vi "Reset Label Strings.vi"(4 "Tick Array":T2, 5 "Right justified":bool, 6 "Range":cluster{"Max X":sgl, "Min X":sgl}, 7 "Which Axis?":T1(ring)=enum."Z Opposite", 8 "error in (no error)":errorcluster, 9 "Inverted?":bool, 10 "Size":u16, 11 "Axis Scene Object in":refnum<vi>) -> (0 "error out":errorcluster, 3 "Axis Scene Object out":refnum<vi>)   [LabVIEW 2017, in "3D Plot.lvclass"]
uses:
  <vilib>/Math Plots/3D Math Plots/3D Plot/3D Plot/3D Plot.lvclass
  <vilib>/Math Plots/3D Math Plots/3D Plot/3D Plot/Typedef/Tick Array.ctl
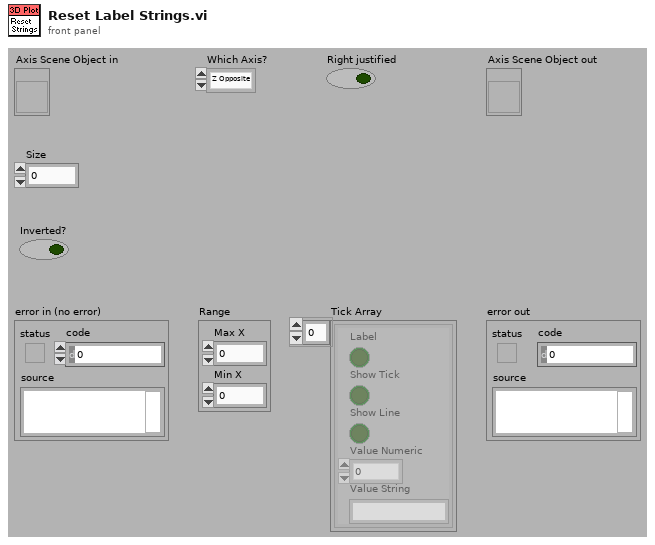
[diagram p1: front panel]
types:
  T1 = enum16{"X", "Y", "Z", "X Opposite", "Y Opposite", "Z Opposite"}
  T2 = typedef "3D Plot.lvclass/Tick Array.ctl" = cluster{"Label":bool, "Show Tick":bool, "Show Line":bool, "Value Numeric":sgl, "Value String":string}[]
  T3 = typedef "LVRGBAColorTypeDef.ctl" = cluster{"Red":sgl, "Green":sgl, "Blue":sgl, "Alpha":sgl}
  T4 = typedef "LV3DPointTypeDef.ctl" = cluster{"X":sgl, "Y":sgl, "Z":sgl}
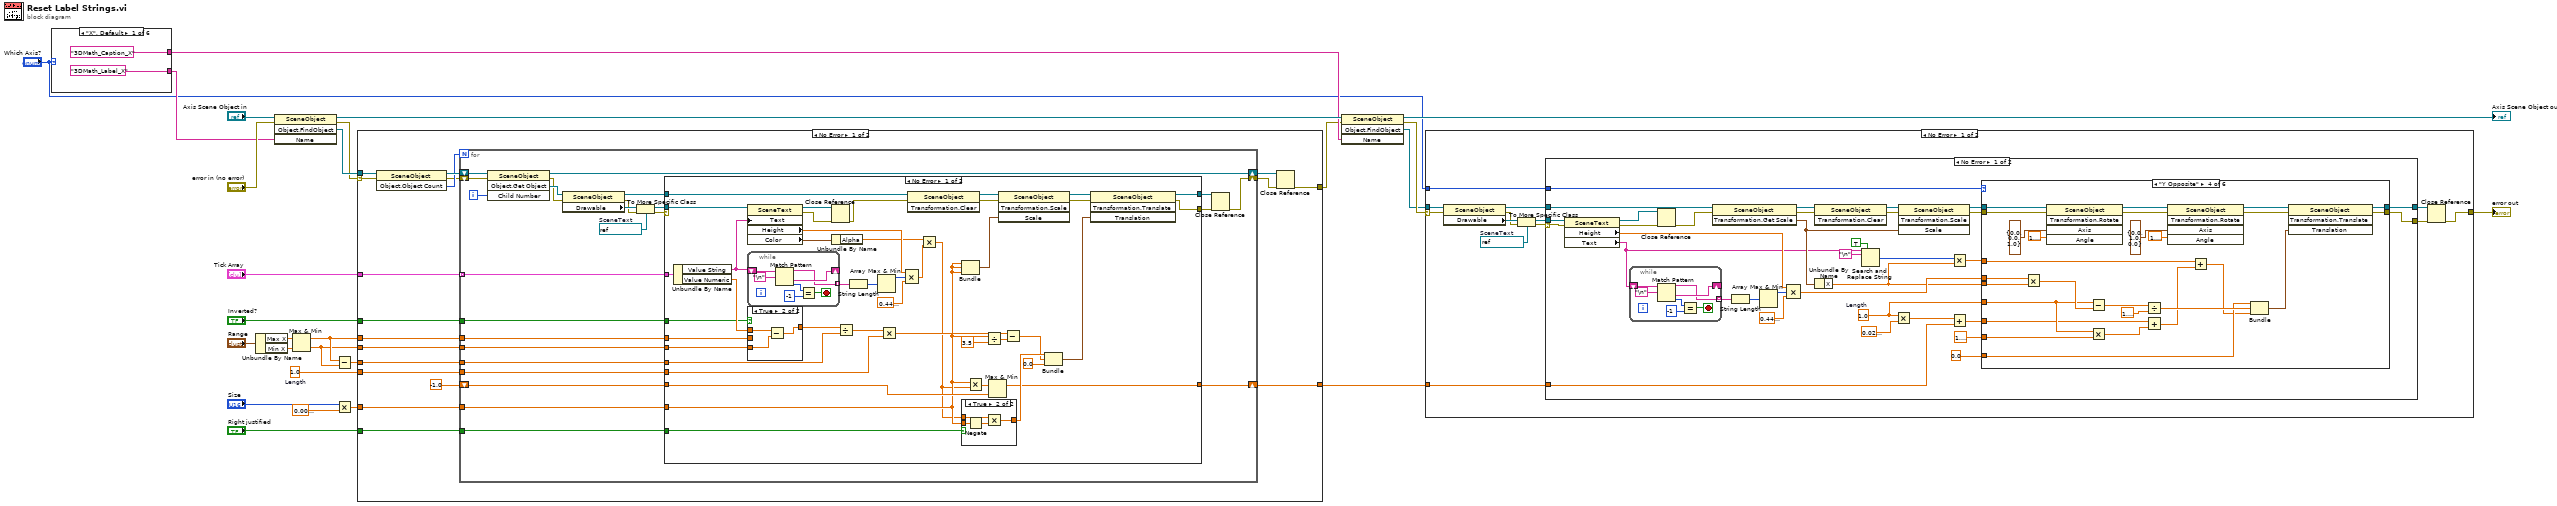
[diagram p0: block diagram]
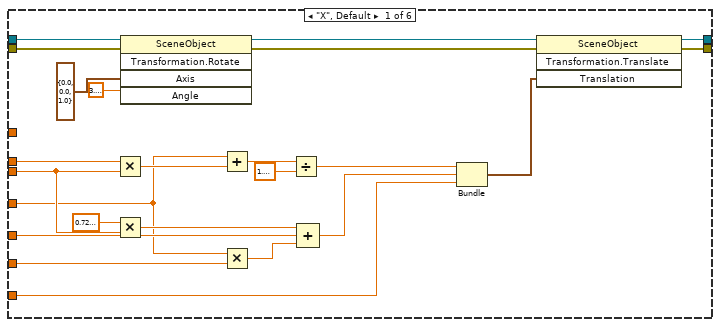
[diagram p2: hidden frame]
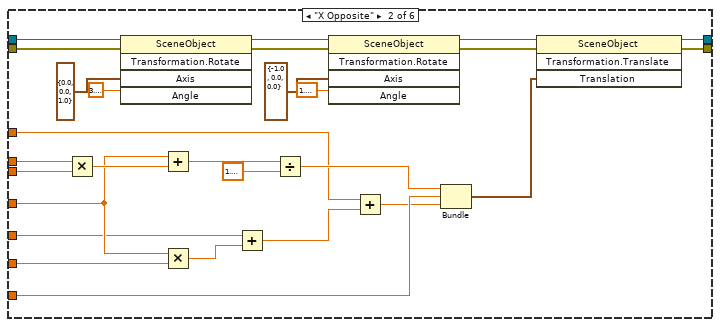
[diagram p3: hidden frame]
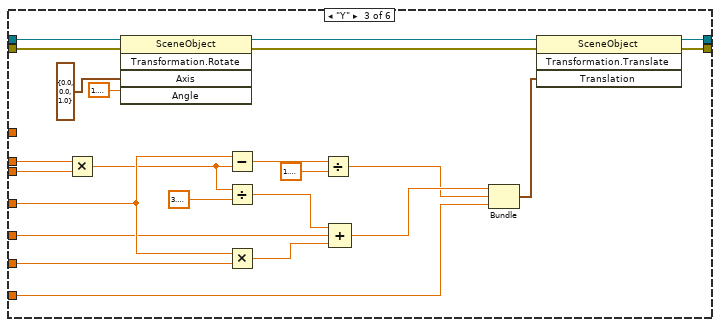
[diagram p4: hidden frame]
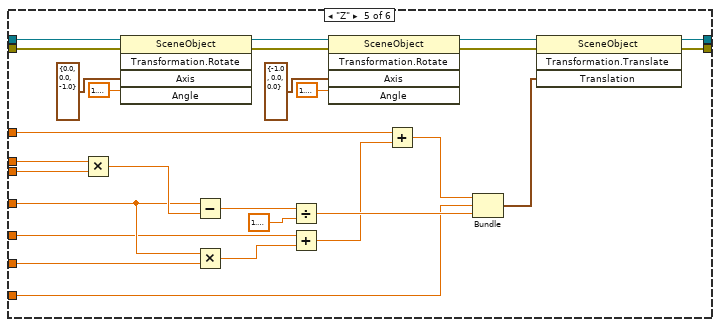
[diagram p5: hidden frame]
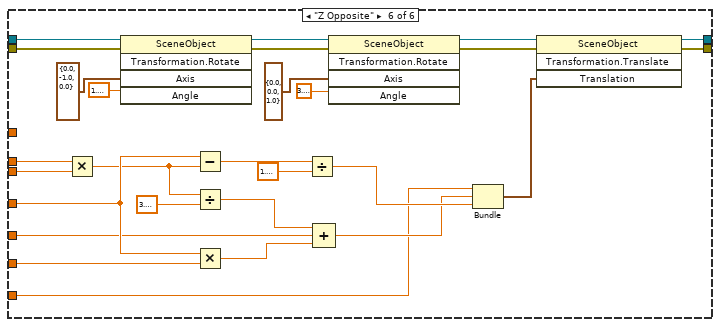
[diagram p6: hidden frame]
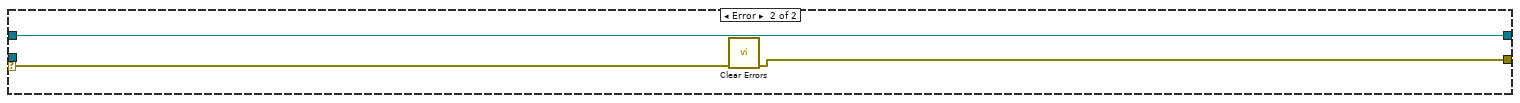
[diagram p7: hidden frame]
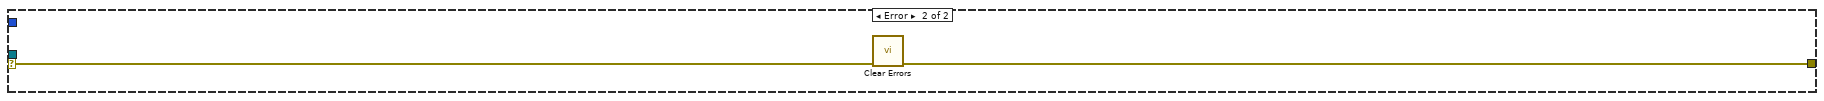
[diagram p8: hidden frame]
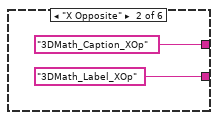
[diagram p9: hidden frame]
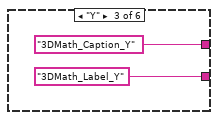
[diagram p10: hidden frame]
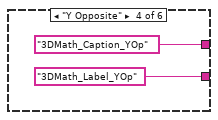
[diagram p11: hidden frame]
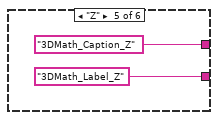
[diagram p12: hidden frame]
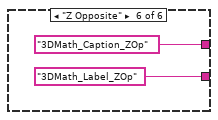
[diagram p13: hidden frame]
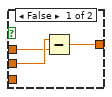
[diagram p14: hidden frame]
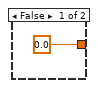
[diagram p15: hidden frame]
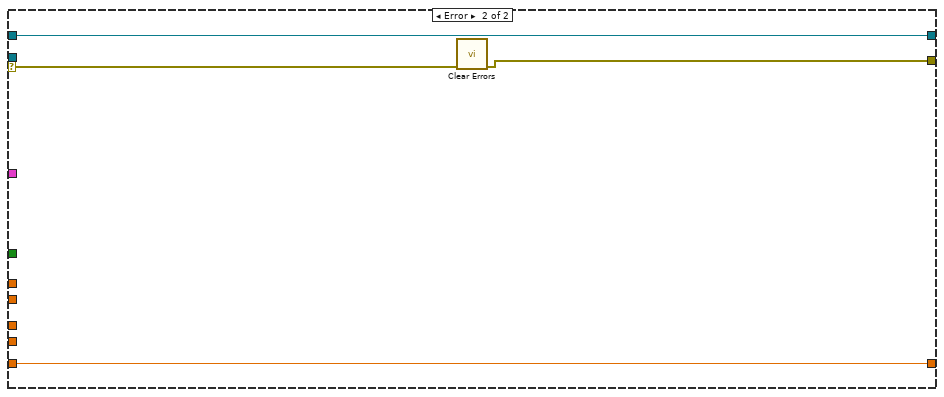
[diagram p16: hidden frame]
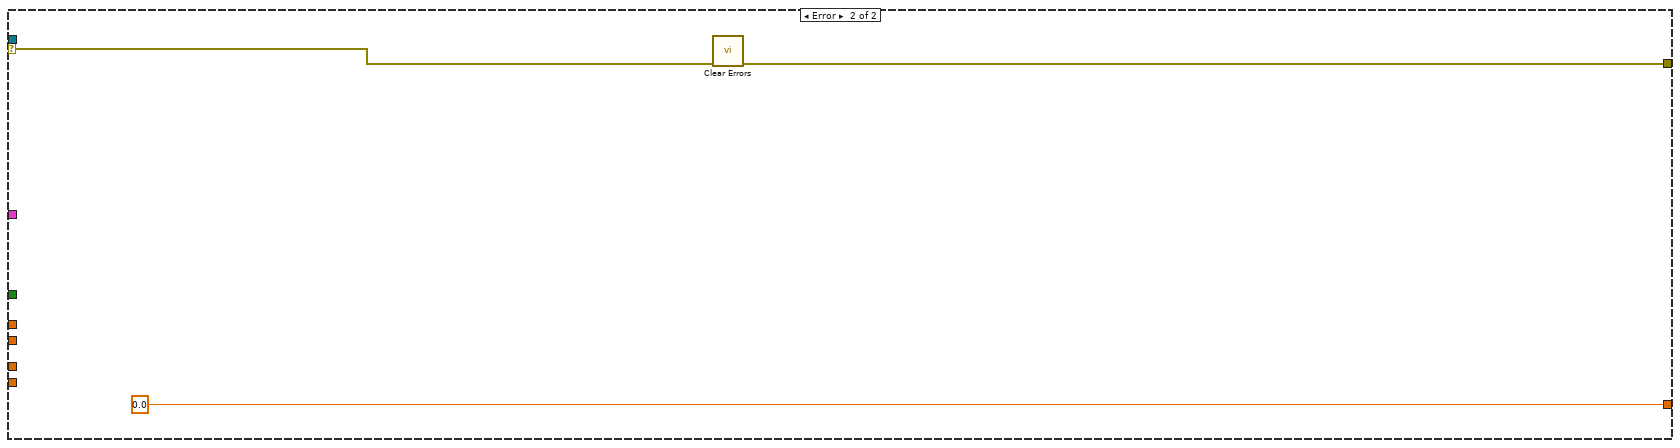
[diagram p17: hidden frame]
diagram:
  w11 = sgl 1.0  # Length
  n1 = case shown="\"X\", Default" "Which Axis?" {
    tunnel: ["3DMath_Label_X" ("Label Object Name") "3DMath_Label_XOp" ("Label Object Name") "3DMath_Label_Y" ("Label Object Name") "3DMath_Label_YOp" ("Label Object Name") "3DMath_Label_Z" ("Label Object Name") "3DMath_Label_ZOp" ("Label Object Name")] -> w9
    tunnel: ["3DMath_Caption_X" "3DMath_Caption_XOp" "3DMath_Caption_Y" "3DMath_Caption_YOp" "3DMath_Caption_Z" "3DMath_Caption_ZOp"] -> w7
    frame "X", Default {
    }
    frame "X Opposite" {
    }
    frame "Y" {
    }
    frame "Y Opposite" {
    }
    frame "Z" {
    }
    frame "Z Opposite" {
    }
  }
  n2 = Unbundle By Name("Range") -> ("Max X"=w18:sgl, "Min X"=w19:sgl)
  n3 = invoke class="SceneObject" method="Object.FindObject"(reference="Axis Scene Object in", error in="error in (no error)", "Name"=w9) -> (reference out=w24:refnum<vi>, error out=w22:errorcluster, "FindObject"=w23:refnum<vi>)  [unwired: 1 in, 1 out]
  n4 = Max & Min(x=w18, y=w19) -> (max(x,y)=w13:sgl, min(x,y)=w12:sgl)
  n5 = Subtract(x=w13, y=w12) -> (x-y=w15:sgl)
  n6 = Multiply(x="Size", y=sgl 0.01) -> (x*y=w10:sgl)
  n7 = case shown="No Error" w22 {
    selector: w22 -> [w57 w150]
    tunnel: w23 -> [w56 _]
    tunnel: [w49 w149] -> w4
    tunnel: "Tick Array" -> [w52 _]
    tunnel: w10 -> [w48 _]
    tunnel: "Right justified" -> [w47 _]
    tunnel: w11 -> [w46 _]
    tunnel: w15 -> [w45 _]
    tunnel: "Inverted?" -> [w44 _]
    tunnel: w13 -> [w43 _]
    tunnel: w12 -> [w42 _]
    tunnel: [w41 sgl 0.0] -> w1
    frame No Error {
      n8 = invoke class="SceneObject" method="Object.Object Count"(reference=w56, error in=w57) -> (reference out=w55:refnum<vi>, error out=w53:errorcluster, "Child Count"=w54:i32)  [unwired: 1 in]
      n9 = for {
        N: w54 -> [_]
        shift-right: [w73] -> w51
        shift-left: w53 -> [w80]
        tunnel: w52 -> [w61] mode=indexing
        shift-right: [w72] -> w50
        shift-left: w55 -> [w82]
        shift-right: [w67] -> w41
        shift-left: sgl -1.0 -> [w66]
        tunnel: w48 -> [w65]
        tunnel: w47 -> [w64]
        tunnel: w46 -> [w63]
        tunnel: w45 -> [w62]
        tunnel: w44 -> [w60]
        tunnel: w43 -> [w59]
        tunnel: w42 -> [w58]
        i -> [w81]
        w78 = refnum<vi> refnum  # SceneText
        n10 = invoke class="SceneObject" method="Object.Get Object"(reference=w82, error in=w80, "Child Number"=w81) -> (reference out=w72:refnum<vi>, error out=w70:errorcluster, "Get Child"=w71:refnum<vi>)  [unwired: 1 in, 1 out]
        n11 = property class="SceneObject"(reference=w71, error in=w70) -> (reference out=w69:refnum<vi>, error out=w76:errorcluster, "Drawable"=w79:refnum<vi>)
        n12 = To More Specific Class(target class=w78, reference=w79, error in=w76) -> (specific class reference=w77:refnum<vi>, error out=w75:errorcluster)
        n13 = case shown="No Error" w75 {
          selector: w75 -> [_ w147]
          tunnel: w77 -> [w123 _]
          tunnel: [w87 w146] -> w74
          tunnel: w69 -> [w94 w145]
          tunnel: [w116 w145] -> w68
          tunnel: [w105 w144] -> w67
          tunnel: w66 -> [w104 w144]
          tunnel: w65 -> [w92 _]
          tunnel: w64 -> [w103 _]
          tunnel: w63 -> [w102 _]
          tunnel: w62 -> [w101 _]
          tunnel: w61 -> [w99 _]
          tunnel: w60 -> [w97 _]
          tunnel: w59 -> [w96 _]
          tunnel: w58 -> [w95 _]
          frame No Error {
            n14 = Unbundle By Name(w99) -> ("Value String"=w100:string, "Value Numeric"=w98:sgl)
            n15 = property class="SceneText"(reference=w123, "Text"=w100) -> (reference out=w125:refnum<vi>, error out=w124:errorcluster, "Height"=w119:sgl, "Color"=w86:T3)  [unwired: 1 in]
            n16 = while {
              shift-right: [w142] -> _
              shift-left: w100 -> [w143]
              tunnel: [w141] -> w120 mode=indexing
              stop <- w139 stop-if-true
              n17 = Match Pattern(string=w143, regular expression="\n") -> (before substring=w141:string, after substring=w142:string, offset past match=w138:i32)  [unwired: 2 out]
              n18 = Equal?(x=w138, y=-1) -> (x = y?=w139:bool)
            }
            n19 = case shown="True" w97 {
              tunnel: [w128 w129] -> w109
              tunnel: w96 -> [w127 _]
              tunnel: w98 -> [w126 w131]
              tunnel: w95 -> [_ w130]
              frame False {
                n20 = Subtract(x=w127, y=w126) -> (x-y=w128:sgl)
              }
              frame True {
                n21 = Subtract(x=w131, y=w130) -> (x-y=w129:sgl)
              }
            }
            n22 = Close Reference(reference=w125, error in (no error)=w124) -> (error out=w90:errorcluster)
            n23 = Unbundle By Name(w86) -> ("Alpha"=w85:sgl)
            n24 = Divide(x=w109, y=w101) -> (x/y=w108:sgl)
            n25 = String Length(string=w120) -> (length=w121:i32[])
            n26 = Array Max & Min(array=w121) -> (max value=w91:i32)  [unwired: 3 out]
            n27 = Multiply(x=w108, y=w102) -> (x*y=w110:sgl)
            n28 = Compound Arithmetic op=MULTIPLY(w119, w91, sgl 0.45 ("y")) -> (w84:sgl)
            n29 = invoke class="SceneObject" method="Transformation.Clear"(reference=w94, error in=w90) -> (reference out=w118:refnum<vi>, error out=w89:errorcluster)  [unwired: 1 in, 1 out]
            n30 = Multiply(x=w85, y=w84) -> (x*y=w83:sgl)
            n31 = Bundle(w92, w92, w92) -> (w93:cluster{sgl, sgl, sgl})  [unwired: 1 out]
            n32 = case shown="True" w103 {
              tunnel: w92 -> [_ w136]
              tunnel: [sgl 0.0 w135] -> w115
              tunnel: w83 -> [_ w134]
              frame False {
              }
              frame True {
                n33 = Negate(x=w136) -> (-x=w133:sgl)
                n34 = Multiply(x=w134, y=w133) -> (x*y=w135:sgl)
              }
            }
            n35 = Multiply(x=w92, y=w83) -> (x*y=w107:sgl)
            n36 = Divide(x=w92, y=sgl 3.5) -> (x/y=w112:sgl)
            n37 = Max & Min(x=w107, y=w104) -> (max(x,y)=w105:sgl)  [unwired: 1 out]
            n38 = invoke class="SceneObject" method="Transformation.Scale"(reference=w118, error in=w89, "Scale"=w93) -> (reference out=w117:refnum<vi>, error out=w88:errorcluster)  [unwired: 1 in, 2 out]
            n39 = Subtract(x=w110, y=w112) -> (x-y=w111:sgl)
            n40 = Bundle(w115, w111, "Y"=sgl 0.0) -> (w106:cluster{sgl, sgl, "Y":sgl})  [unwired: 1 out]
            n41 = invoke class="SceneObject" method="Transformation.Translate"(reference=w117, error in=w88, "Translation"=w106) -> (reference out=w116:refnum<vi>, error out=w87:errorcluster)  [unwired: 1 in, 2 out]
          }
          frame Error {
            n42 = call <vilib>:"Clear Errors.vi"("error in (no error)"=w147) -> ("error out"=w146:errorcluster)  [unwired: 5 in, 1 out]
          }
        }
        n43 = Close Reference(reference=w68, error in (no error)=w74) -> (error out=w73:errorcluster)
      }
      n44 = Close Reference(reference=w50, error in (no error)=w51) -> (error out=w49:errorcluster)
    }
    frame Error {
      n45 = call <vilib>:"Clear Errors.vi"("error in (no error)"=w150) -> ("error out"=w149:errorcluster)  [unwired: 5 in, 1 out]
    }
  }
  n46 = invoke class="SceneObject" method="Object.FindObject"(reference=w24, error in=w4, "Name"=w7) -> (reference out=→"Axis Scene Object out":refnum<vi>, error out=w6:errorcluster, "FindObject"=w5:refnum<vi>)  [unwired: 1 in, 1 out]
  n47 = case shown="No Error" w6 {
    selector: w6 -> [w158 w364]
    tunnel: w5 -> [w159 _]
    tunnel: [w153 w363] -> w3
    tunnel: "Which Axis?" -> [w161 _]
    tunnel: w1 -> [w160 _]
    frame No Error {
      w163 = refnum<vi> refnum  # SceneText
      n48 = property class="SceneObject"(reference=w159, error in=w158) -> (reference out=w156:refnum<vi>, error out=w152:errorcluster, "Drawable"=w157:refnum<vi>)
      n49 = To More Specific Class(target class=w163, reference=w157, error in=w152) -> (specific class reference=w162:refnum<vi>, error out=w151:errorcluster)
      n50 = case shown="No Error" w151 {
        selector: w151 -> [w164 w362]
        tunnel: w162 -> [w198 _]
        tunnel: w161 -> [w193 _]
        tunnel: w160 -> [w186 _]
        tunnel: w156 -> [w175 w360]
        tunnel: [w172 w360] -> w155
        tunnel: [w171 w361] -> w154
        frame No Error {
          w187 = sgl 1.0  # Length
          n51 = property class="SceneText"(reference=w198, error in=w164) -> (reference out=w178:refnum<vi>, error out=w177:errorcluster, "Height"=w184:sgl, "Text"=w165:string)
          n52 = while {
            shift-right: [w358] -> _
            shift-left: w165 -> [w359]
            tunnel: [w357] -> w196 mode=indexing
            stop <- w355 stop-if-true
            n53 = Match Pattern(string=w359, regular expression="\n") -> (before substring=w357:string, after substring=w358:string, offset past match=w354:i32)  [unwired: 2 out]
            n54 = Equal?(x=w354, y=-1) -> (x = y?=w355:bool)
          }
          n55 = Close Reference(reference=w178, error in (no error)=w177) -> (error out=w176:errorcluster)
          n56 = invoke class="SceneObject" method="Transformation.Get Scale"(reference=w175, error in=w176) -> (reference out=w174:refnum<vi>, error out=w168:errorcluster, "Transformation.Get Scale"=w169:T4)  [unwired: 1 in]
          n57 = String Length(string=w196) -> (length=w195:i32[])
          n58 = Array Max & Min(array=w195) -> (max value=w197:i32)  [unwired: 3 out]
          n59 = Compound Arithmetic op=MULTIPLY(w184, w197, sgl 0.45 ("y")) -> (w185:sgl)
          n60 = invoke class="SceneObject" method="Transformation.Clear"(reference=w174, error in=w168) -> (reference out=w173:refnum<vi>, error out=w167:errorcluster)  [unwired: 1 in, 1 out]
          n61 = Unbundle By Name(w169) -> ("X"=w180:sgl)
          n62 = Search and Replace String(replace all?=TRUE ("replace all? (F)"), input string=w165, search string="\n") -> (number of replacements=w181:i32)  [unwired: 5 in, 3 out]
          n63 = Multiply(x=w187, y=sgl 0.03) -> (x*y=w188:sgl)
          n64 = invoke class="SceneObject" method="Transformation.Scale"(reference=w173, error in=w167, "Scale"=w169) -> (reference out=w170:refnum<vi>, error out=w166:errorcluster)  [unwired: 1 in, 2 out]
          n65 = Multiply(x=w181, y=w180) -> (x*y=w179:sgl)
          n66 = Add(x=w188, y=w186) -> (x+y=w190:sgl)
          n67 = case shown="\"Y Opposite\"" w193 {
            tunnel: w166 -> [w199 w222 w249 w272 w299 w326]
            tunnel: w185 -> [w221 w234 w263 w285 w311 w340]
            tunnel: w170 -> [w200 w223 w250 w273 w300 w327]
            tunnel: [w220 w230 w261 w280 w306 w336] -> w171
            tunnel: [w218 w229 w262 w281 w307 w337] -> w172
            tunnel: w187 -> [w205 w232 w259 w283 w309 w338]
            tunnel: w190 -> [w217 w231 w254 w282 w308 w332]
            tunnel: w180 -> [w216 w233 w260 w284 w310 w339]
            tunnel: sgl 1.1 ("y") -> [w204 w228 w253 w279 w305 w330]
            tunnel: sgl 0.0 ("x+y") -> [w202 w227 w252 w276 w304 w329]
            tunnel: w179 -> [_ w225 _ w278 w303 _]
            frame "X", Default {
              n68 = Multiply(x=w221, y=w216) -> (x*y=w212:sgl)
              n69 = Multiply(x=sgl 0.72, y=w216) -> (x*y=w207:sgl)
              n70 = invoke class="SceneObject" method="Transformation.Rotate"(reference=w200, error in=w199, "Axis"=cluster{"X":sgl, "Y":sgl, "Z":sgl} {"X"=0.0, "Y"=0.0, "Z"=1.0}, "Angle"=sgl 3.1415927) -> (reference out=w208:refnum<vi>, error out=w219:errorcluster)  [unwired: 1 in, 3 out]
              n71 = Add(x=w205, y=w212) -> (x+y=w213:sgl)
              n72 = Multiply(x=w205, y=w204) -> (x*y=w203:sgl)
              n73 = Divide(x=w213, y=sgl 1.9) -> (x/y=w215:sgl)
              n74 = Compound Arithmetic op=ADD(w207, w217, w203) -> (w201:sgl)
              n75 = Bundle(w215, w201, "x+y"=w202) -> (w211:cluster{sgl, sgl, "x+y":sgl})  [unwired: 1 out]
              n76 = invoke class="SceneObject" method="Transformation.Translate"(reference=w208, error in=w219, "Translation"=w211) -> (reference out=w218:refnum<vi>, error out=w220:errorcluster)  [unwired: 1 in, 2 out]
            }
            frame "X Opposite" {
              n77 = Multiply(x=w234, y=w233) -> (x*y=w248:sgl)
              n78 = invoke class="SceneObject" method="Transformation.Rotate"(reference=w223, error in=w222, "Axis"=cluster{"X":sgl, "Y":sgl, "Z":sgl} {"X"=0.0, "Y"=0.0, "Z"=1.0}, "Angle"=sgl 3.1415927) -> (reference out=w244:refnum<vi>, error out=w236:errorcluster)  [unwired: 1 in, 3 out]
              n79 = Add(x=w232, y=w248) -> (x+y=w247:sgl)
              n80 = Multiply(x=w232, y=w228) -> (x*y=w245:sgl)
              n81 = Add(x=w231, y=w245) -> (x+y=w226:sgl)
              n82 = Divide(x=w247, y=sgl 1.9) -> (x/y=w237:sgl)
              n83 = invoke class="SceneObject" method="Transformation.Rotate"(reference=w244, error in=w236, "Axis"=cluster{"X":sgl, "Y":sgl, "Z":sgl} {"X"=-1.0, "Y"=0.0, "Z"=0.0}, "Angle"=sgl 1.5707964) -> (reference out=w238:refnum<vi>, error out=w235:errorcluster)  [unwired: 1 in, 3 out]
              n84 = Add(x=w225, y=w226) -> (x+y=w224:sgl)
              n85 = Bundle(w237, "x+y"=w227, w224) -> (w243:cluster{sgl, "x+y":sgl, sgl})  [unwired: 1 out]
              n86 = invoke class="SceneObject" method="Transformation.Translate"(reference=w238, error in=w235, "Translation"=w243) -> (reference out=w229:refnum<vi>, error out=w230:errorcluster)  [unwired: 1 in, 2 out]
            }
            frame "Y" {
              n87 = Multiply(x=w263, y=w260) -> (x*y=w256:sgl)
              n88 = invoke class="SceneObject" method="Transformation.Rotate"(reference=w250, error in=w249, "Axis"=cluster{"X":sgl, "Y":sgl, "Z":sgl} {"X"=0.0, "Y"=0.0, "Z"=1.0}, "Angle"=sgl 1.5707964) -> (reference out=w269:refnum<vi>, error out=w271:errorcluster)  [unwired: 1 in, 3 out]
              n89 = Subtract(x=w259, y=w256) -> (x-y=w264:sgl)
              n90 = Divide(x=w256, y=sgl 3.7) -> (x/y=w257:sgl)
              n91 = Multiply(x=w259, y=w253) -> (x*y=w251:sgl)
              n92 = Divide(x=w264, y=sgl 1.8) -> (x/y=w258:sgl)
              n93 = Compound Arithmetic op=ADD(w257, w254, w251) -> (w270:sgl)
              n94 = Bundle(w270, w258, "x+y"=w252) -> (w266:cluster{sgl, sgl, "x+y":sgl})  [unwired: 1 out]
              n95 = invoke class="SceneObject" method="Transformation.Translate"(reference=w269, error in=w271, "Translation"=w266) -> (reference out=w262:refnum<vi>, error out=w261:errorcluster)  [unwired: 1 in, 2 out]
            }
            frame "Y Opposite" {
              n96 = Multiply(x=w285, y=w284) -> (x*y=w286:sgl)
              n97 = invoke class="SceneObject" method="Transformation.Rotate"(reference=w273, error in=w272, "Axis"=cluster{"X":sgl, "Y":sgl, "Z":sgl} {"X"=0.0, "Y"=0.0, "Z"=1.0}, "Angle"=sgl 1.5707964) -> (reference out=w290:refnum<vi>, error out=w297:errorcluster)  [unwired: 1 in, 3 out]
              n98 = Subtract(x=w283, y=w286) -> (x-y=w287:sgl)
              n99 = Multiply(x=w283, y=w279) -> (x*y=w289:sgl)
              n100 = Divide(x=w287, y=sgl 1.8) -> (x/y=w277:sgl)
              n101 = Add(x=w282, y=w289) -> (x+y=w275:sgl)
              n102 = invoke class="SceneObject" method="Transformation.Rotate"(reference=w290, error in=w297, "Axis"=cluster{"X":sgl, "Y":sgl, "Z":sgl} {"X"=0.0, "Y"=1.0, "Z"=0.0}, "Angle"=sgl 1.5707964) -> (reference out=w295:refnum<vi>, error out=w298:errorcluster)  [unwired: 1 in, 3 out]
              n103 = Add(x=w278, y=w275) -> (x+y=w274:sgl)
              n104 = Bundle("x+y"=w276, w277, w274) -> (w291:cluster{"x+y":sgl, sgl, sgl})  [unwired: 1 out]
              n105 = invoke class="SceneObject" method="Transformation.Translate"(reference=w295, error in=w298, "Translation"=w291) -> (reference out=w281:refnum<vi>, error out=w280:errorcluster)  [unwired: 1 in, 2 out]
            }
            frame "Z" {
              n106 = Multiply(x=w311, y=w310) -> (x*y=w312:sgl)
              n107 = invoke class="SceneObject" method="Transformation.Rotate"(reference=w300, error in=w299, "Axis"=cluster{"X":sgl, "Y":sgl, "Z":sgl} {"X"=0.0, "Y"=0.0, "Z"=-1.0}, "Angle"=sgl 1.5707964) -> (reference out=w316:refnum<vi>, error out=w324:errorcluster)  [unwired: 1 in, 3 out]
              n108 = Subtract(x=w309, y=w312) -> (x-y=w313:sgl)
              n109 = Multiply(x=w309, y=w305) -> (x*y=w315:sgl)
              n110 = Divide(x=w313, y=sgl 1.8) -> (x/y=w323:sgl)
              n111 = Add(x=w308, y=w315) -> (x+y=w302:sgl)
              n112 = invoke class="SceneObject" method="Transformation.Rotate"(reference=w316, error in=w324, "Axis"=cluster{"X":sgl, "Y":sgl, "Z":sgl} {"X"=-1.0, "Y"=0.0, "Z"=0.0}, "Angle"=sgl 1.5707964) -> (reference out=w321:refnum<vi>, error out=w325:errorcluster)  [unwired: 1 in, 3 out]
              n113 = Add(x=w303, y=w302) -> (x+y=w301:sgl)
              n114 = Bundle(w301, "x+y"=w304, w323) -> (w317:cluster{sgl, "x+y":sgl, sgl})  [unwired: 1 out]
              n115 = invoke class="SceneObject" method="Transformation.Translate"(reference=w321, error in=w325, "Translation"=w317) -> (reference out=w307:refnum<vi>, error out=w306:errorcluster)  [unwired: 1 in, 2 out]
            }
            frame "Z Opposite" {
              n116 = Multiply(x=w340, y=w339) -> (x*y=w333:sgl)
              n117 = invoke class="SceneObject" method="Transformation.Rotate"(reference=w327, error in=w326, "Axis"=cluster{"X":dbl, "Y":dbl, "Z":dbl} {"X"=0.0, "Y"=-1.0, "Z"=0.0}, "Angle"=sgl 1.5707964) -> (reference out=w345:refnum<vi>, error out=w342:errorcluster)  [unwired: 1 in, 3 out]
              n118 = Subtract(x=w338, y=w333) -> (x-y=w352:sgl)
              n119 = Divide(x=w333, y=sgl 3.7) -> (x/y=w334:sgl)
              n120 = Multiply(x=w338, y=w330) -> (x*y=w328:sgl)
              n121 = Divide(x=w352, y=sgl 1.8) -> (x/y=w348:sgl)
              n122 = Compound Arithmetic op=ADD(w334, w332, w328) -> (w331:sgl)
              n123 = invoke class="SceneObject" method="Transformation.Rotate"(reference=w345, error in=w342, "Axis"=cluster{"X":dbl, "Y":dbl, "Z":dbl} {"X"=0.0, "Y"=0.0, "Z"=1.0}, "Angle"=sgl 3.1415927) -> (reference out=w344:refnum<vi>, error out=w341:errorcluster)  [unwired: 1 in, 3 out]
              n124 = Bundle("x+y"=w329, w331, w348) -> (w350:cluster{"x+y":sgl, sgl, sgl})  [unwired: 1 out]
              n125 = invoke class="SceneObject" method="Transformation.Translate"(reference=w344, error in=w341, "Translation"=w350) -> (reference out=w337:refnum<vi>, error out=w336:errorcluster)  [unwired: 1 in, 2 out]
            }
          }
        }
        frame Error {
          n126 = call <vilib>:"Clear Errors.vi"("error in (no error)"=w362) -> ("error out"=w361:errorcluster)  [unwired: 5 in, 1 out]
        }
      }
      n127 = Close Reference(reference=w155, error in (no error)=w154) -> (error out=w153:errorcluster)
    }
    frame Error {
      n128 = call <vilib>:"Clear Errors.vi"("error in (no error)"=w364) -> ("error out"=w363:errorcluster)  [unwired: 5 in, 1 out]
    }
  }
  "error out" <- w3
